vi "splash.vi"(11 "Chain IN":bool) -> (3 "Chain OUT":bool)   [LabVIEW 2010, in "LASA Beta.lvrbt"]
uses:
  LASA Beta.lvrbt
  <vilib>/NXT/Block Support/NXT_FileStatusCodes.ctl
  <vilib>/NXT/Dual Mode Library/Display/drawPicture.vi
  <vilib>/NXT/Dual Mode Library/Display/drawText.vi
  <vilib>/NXT/Dual Mode Library/Display/clearDisplay.vi
  <vilib>/NXT/Dual Mode Library/Waits/Wait_Num(msec).vi
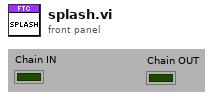
[diagram p1: front panel]
types:
  T1 = typedef "LVHSConnector.ctl" = cluster{"Hardware":string, "Flattened String":string}
  T2 = typedef "NXT_FileStatusCodes.ctl" = u16
  T3 = typedef "SequenceBoolean.ctl" = bool
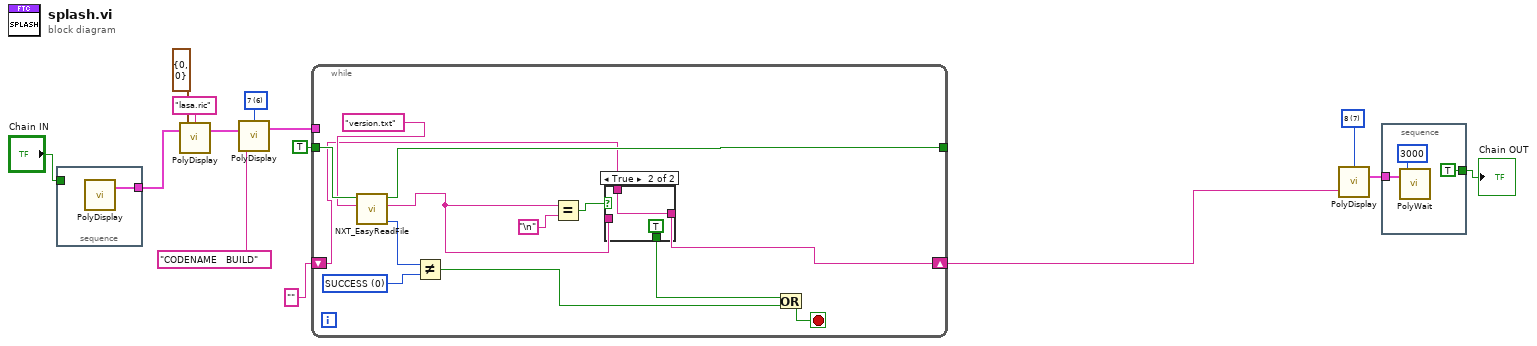
[diagram p0: block diagram]
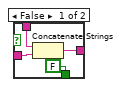
[diagram p2: hidden frame]
diagram:
  w5 = i16 6 items=["1", "2", "3", "4", "5", "6", "7", "8"] ("Line")
  w11 = i16 7 items=["1", "2", "3", "4", "5", "6", "7", "8"] ("Line")
  n1 = stacked-sequence {
    tunnel: "Chain IN" -> [_]
    tunnel: [w15] -> w3
    frame #0 {
      n2 = call-poly <vilib>:"PolyDisplay.vi"() -> ("NXT"=w15:T1)  [unwired: 4 in]
    }
  }
  n3 = call-poly <vilib>:"PolyDisplay.vi"("Origin"=cluster{"X":i16, "Y":i16} {"X"=0, "Y"=0}, "NXT"=w3, "Filename (*.ric)"="lasa.ric") -> ("NXT"=w8:T1)  [unwired: 1 in]
  n4 = call-poly <vilib>:"PolyDisplay.vi"("Text"="CODENAME   BUILD", "NXT"=w8, "Line"=w5) -> ("NXT"=w6:T1)  [unwired: 1 in]
  n5 = while {
    tunnel: TRUE -> [w28]
    tunnel: [w26] -> _
    shift-right: [w22] -> w1
    shift-left: "" -> [w23]
    tunnel: w6 -> [_]
    stop <- w19 stop-if-true
    w24 = T2 0 items=["SUCCESS"=0, "NO_HANDLES"=33024, "NO_FILES"=33536, "PARTIAL_WRITE"=33792, "EOF"=34048, "FILE_NOT_FOUND"=34560, "FILE_CLOSED"=34816, "NO_LINEAR_SPACE"=35072, "GENERIC_ERROR"=35328, "FILE_BUSY"=35584, "NO_WRITE_BUFFERS"=35840, "ILLEGAL_APPEND"=36096, "FILE_FULL"=36352, "FILE_EXISTS"=36608, "ILLEGAL_FILE_NAME"=37376, "ILLEGAL_HANDLE"=37632] ("y")
    n6 = call <vilib>:"NXT_EasyReadFile.vi"("Filename"="version.txt", "Sequence Flow in"=w28) -> ("Error out"=w25:T2, "Text"=w20:string, "Sequence Flow out"=w26:T3)  [unwired: 6 in, 1 out]
    n7 = Not Equal?(x=w25, y=w24) -> (x != y?=w17:bool)
    n8 = Equal?(x=w20, y="\n" ("Line Feed Constant")) -> (x = y?=w21:bool)
    n9 = case shown="True" w21 {
      tunnel: w20 -> [w32 _]
      tunnel: w23 -> [w31 w34]
      tunnel: [w30 w34] -> w22
      tunnel: [FALSE TRUE] -> w18
      frame False {
        n10 = Concatenate Strings(w31, w32) -> (w30:string)
      }
      frame True {
      }
    }
    n11 = Or(x=w18, y=w17) -> (x .or. y?=w19:bool)
  }
  n12 = call-poly <vilib>:"PolyDisplay.vi"("Text"=w1, "Line"=w11) -> ("NXT"=w10:T1)  [unwired: 2 in]
  n13 = stacked-sequence {
    tunnel: w10 -> [w37]
    tunnel: [TRUE] -> w2
    frame #0 {
      n14 = call-poly <vilib>:"PolyWait.vi"("Time (100 msec)"=u32 3000, "NXT"=w37) -> ()  [unwired: 2 in, 1 out]
    }
  }
  "Chain OUT" <- w2
